vi "MC_Init_Selections.vi"(8 "error in (no error)":errorcluster, 11 "MCin":refnum<vi>) -> (0 "error out":errorcluster, 3 "MCout":refnum<vi>)   [LabVIEW 2013]
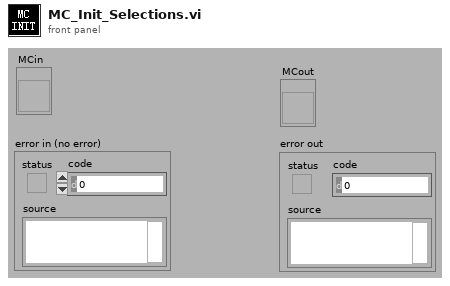
[diagram p1: front panel]
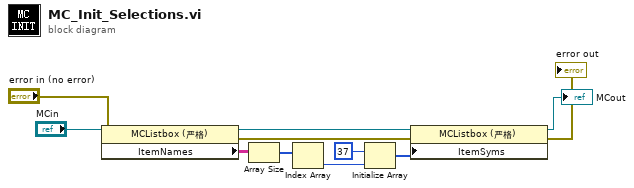
[diagram p0: block diagram]
diagram:
  n1 = property on="属性节点" class="MCListbox (严格)"(reference="MCin", error in="error in (no error)") -> (reference out=w5:refnum<vi>, error out=w4:errorcluster, "ItemNames"=w11:string[][])
  n2 = Array Size(array=w11) -> (size(s)=w10:i32[])
  n3 = Index Array(array=w10) -> (element=w9:i32)  [unwired: 1 in]
  n4 = Initialize Array(37, w9) -> (w7:i32[])
  n5 = property on="属性节点" class="MCListbox (严格)"(reference=w5, error in=w4, "ItemSyms"=w7) -> (reference out=→"MCout":refnum<vi>, error out=→"error out":errorcluster)
